vi "Property Tree_Update Value.vi"(8 "error in":errorcluster, 11 "Tree Ref Array Out":refnum<vi>[](array[refnum])) -> (0 "error out":errorcluster)   [LabVIEW 2023]
doc: "Update tree values and symbols after redrawing tree when filtering."
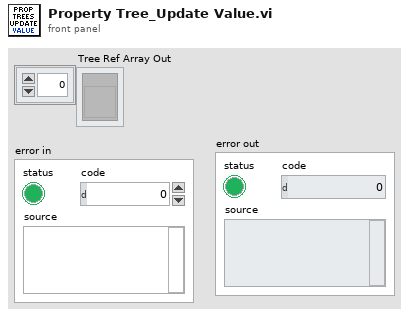
[diagram p1: front panel]
types:
  T1 = enum16{"Init", "Read", "Remove", "Remove or Append", "Append", "Append If New"}
  T2 = cluster{"Tag":string, "Read":bool, "Write":bool, "New":bool}[]
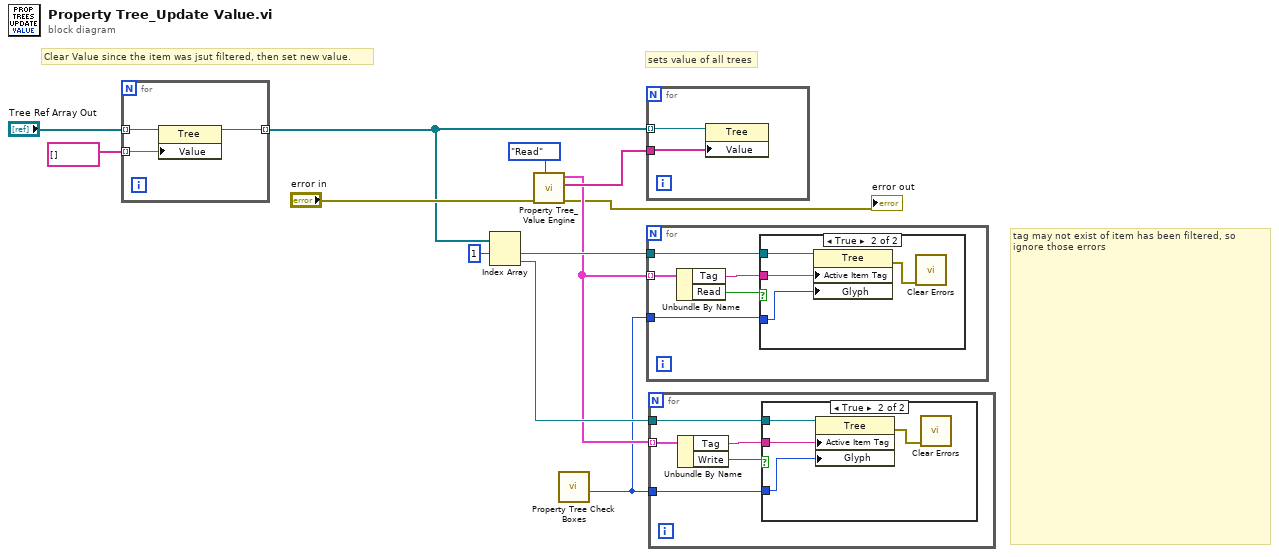
[diagram p0: block diagram]
diagram:
  # "Clear Value since the item was jsut filtered, then set new value."
  # "tag may not exist of item has been filtered, so ignore those errors"
  # "sets value of all trees"
  n1 = for {
    tunnel: "Tree Ref Array Out" -> [w15] mode=indexing
    tunnel: [w14] -> w2 mode=indexing
    tunnel: string[] [] ("Tag Array") -> [w13] mode=indexing
    n2 = property class="Tree"(reference=w15, "Value"=w13) -> (reference out=w14:refnum<vi>)  [unwired: 1 in, 1 out]
  }
  n3 = Index Array(array=w2, index #1=1 ("index")) -> (element #1=w8:refnum<vi>, element #2=w7:refnum<vi>)  [unwired: 1 in]
  n4 = call "Property Tree_Value Engine.vi"("Save Action"=T1."Read" ("Action"), "Error In"="error in") -> ("Error Out"=→"error out":errorcluster, "Tag Array"=w11:string[], "Property Array Out"=w6:T2)  [unwired: 7 in]
  n5 = call "Property Tree Check Boxes.vi"() -> ("Checked"=w5:i32)  [unwired: 9 in, 2 out]
  n6 = for {
    tunnel: w11 -> [w16]
    tunnel: w2 -> [w17] mode=indexing
    n7 = property class="Tree"(reference=w17, "Value"=w16) -> ()  [unwired: 1 in, 2 out]
  }
  n8 = for {
    tunnel: w6 -> [w22] mode=indexing
    tunnel: w5 -> [w20]
    tunnel: w8 -> [w18]
    n9 = Unbundle By Name(w22) -> ("Tag"=w21:string, "Read"=w19:bool)
    n10 = case shown="True" w19 {
      tunnel: w21 -> [_ w26]
      tunnel: w20 -> [_ w25]
      tunnel: w18 -> [_ w24]
      frame False {
      }
      frame True {
        n11 = property class="Tree"(reference=w24, "Active Item Tag"=w26, "Glyph"=w25) -> (error out=w23:errorcluster)  [unwired: 1 in, 1 out]
        n12 = call <vilib>:"Clear Errors.vi"("error in (no error)"=w23) -> ()  [unwired: 5 in, 2 out]
      }
    }
  }
  n13 = for {
    tunnel: w6 -> [w31] mode=indexing
    tunnel: w5 -> [w29]
    tunnel: w7 -> [w27]
    n14 = Unbundle By Name(w31) -> ("Tag"=w30:string, "Write"=w28:bool)
    n15 = case shown="True" w28 {
      tunnel: w30 -> [_ w35]
      tunnel: w29 -> [_ w34]
      tunnel: w27 -> [_ w33]
      frame False {
      }
      frame True {
        n16 = property class="Tree"(reference=w33, "Active Item Tag"=w35, "Glyph"=w34) -> (error out=w32:errorcluster)  [unwired: 1 in, 1 out]
        n17 = call <vilib>:"Clear Errors.vi"("error in (no error)"=w32) -> ()  [unwired: 5 in, 2 out]
      }
    }
  }
